vi "BundleAutoSpotData.vi"(2 "auto":bool, 3 "notes 2":refnum<vi>, 4 "already x spots":i16, 5 "Enum":enum16{"1st sort", "Display", "Get"}(ring)) -> (1 "Spots out":T1[](array[typedef]) {"F2-Value overall" format="%.2f"; "tauerror" format="%.2f"; "Lifetime[ns]" format="%.2f"; "F2-Value TAC" format="%.2f"})   [LabVIEW 2009]
uses:
  spotproperties.ctl
  <vilib>/vision/NI_Vision_Development_Module.lvlib
panel:
  in  "draw?":bool
  in  "notes":string
  out "F2-Value overall":sgl format="%.2f"
  in  "Ring":u16(ring) items=["linear y-axis", "log y-axis"]
  in  "stop":bool
  out "TAC intensity":u32[](array[numeric])
  out "overall intensity":u32[](array[numeric])
  out "tauerror [ns]":dbl[](array[numeric]) format="%.2f"
  out "Lifetime [ns]":ext[](array[numeric]) format="%.2f"
  out "F2-Value TAC":dbl format="%.2f"
  in  "SpotNo.":u16 min=1 max=74
  out "Decays":u32[][](graph)
  # "S"
  # "S"
  # "S"
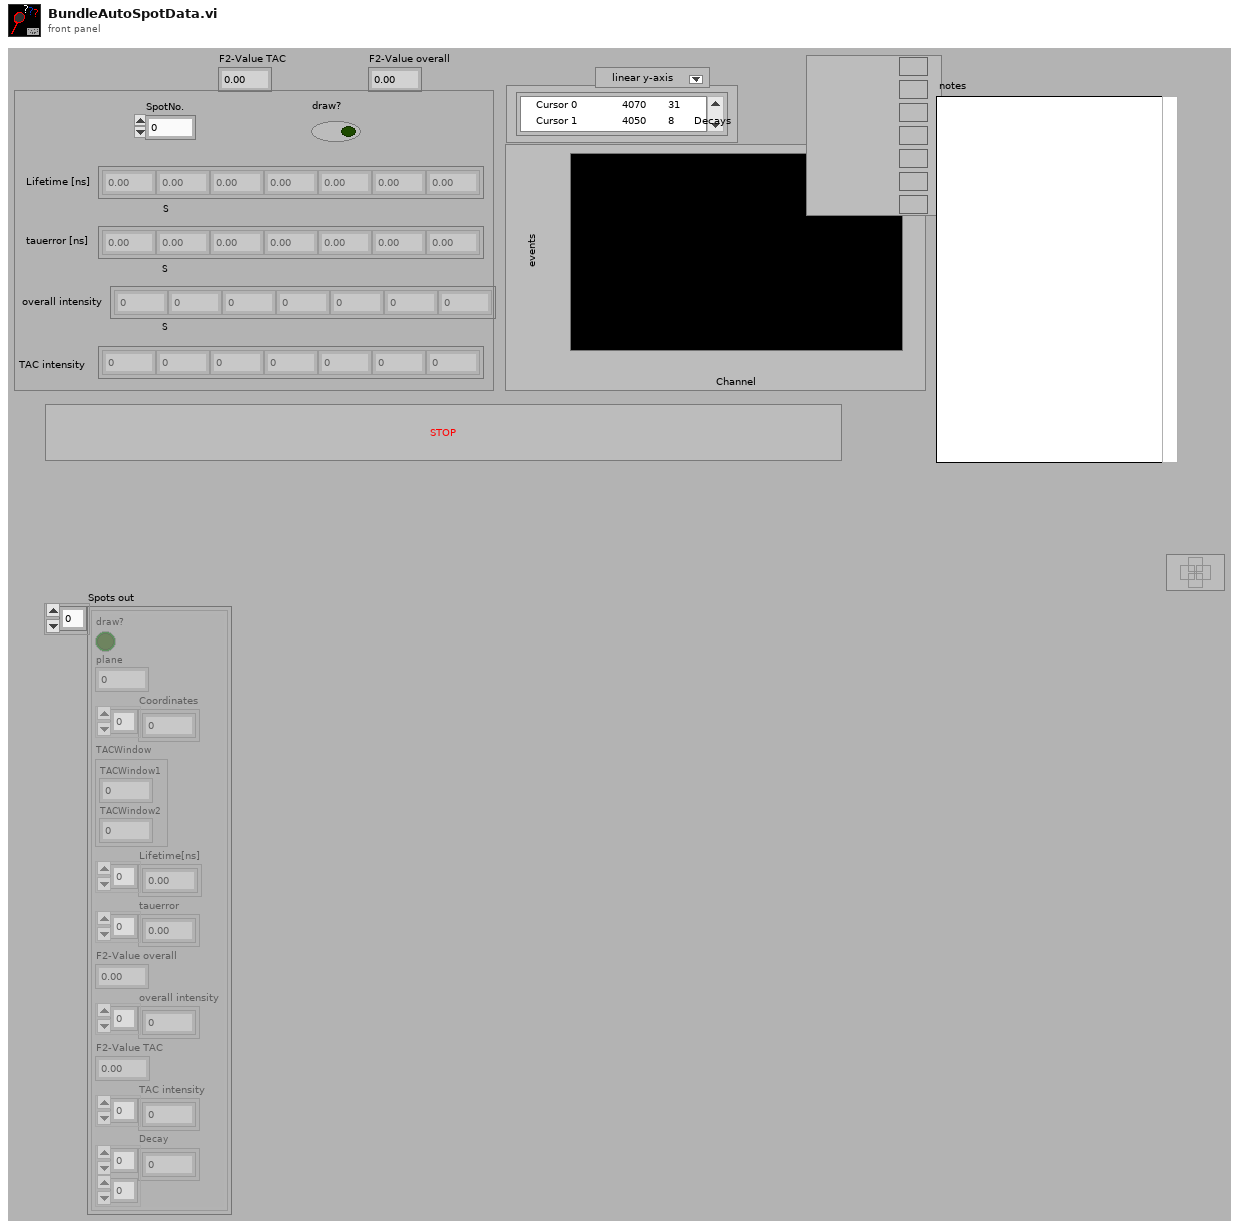
[diagram p1: front panel]
types:
  T1 = typedef "spotproperties.ctl" = cluster{"draw?":bool, "plane":u32, "Coordinates":i32[], "TACWindow":cluster{"TACWindow1":i32, "TACWindow2":i32}, "Lifetime[ns]":ext[], "tauerror":dbl[], "F2-Value overall":dbl, "overall intensity":u32[], "F2-Value TAC":dbl, "TAC intensity":u32[], "Decay":u32[][]}
  T2 = enum16{"Ini", "Get", "Set", "Refresh", "dump", "move", "name"}
  T3 = typedef "Settings.ctl" = cluster{"threshold":cluster{"max":u32, "min":u32}, "RGB or false color":bool, "16bit":bool, "log/lin axis":u16, "spotsize button":bool, "Pixelsize":u16, "autoscale x":bool, "autoscale y":bool, "correlation":bool, "ADC-Resolution":i32, "F2-lifetime":cluster{"display tau":bool, "display F2":bool, "Palette Number lifetime":enum32{"Gray", "Binary", "Gradient", "Rainbow", "Temperature"}, "Palette Number F2":enum32{"Gray", "Binary", "Gradient", "Rainbow", "Temperature"}, "max tau-Value":dbl, "min tau-Value":dbl, "max F2-Value":dbl, "min F2-Value":dbl}, "TAC-Window 1":u16, "TAC-Window 2":u16, "false color palette":cluster{"1":u32, "2":u32, "3":u32, "4":u32, "5":u32, "6":u32, "7":u32, "8":u32, "8 2":u32, "8 3":u32, "8 4":u32, "8 5":u32}, "rebinning":dbl}
  T4 = typedef "IMAQ Image.ctl" = refnum<image>
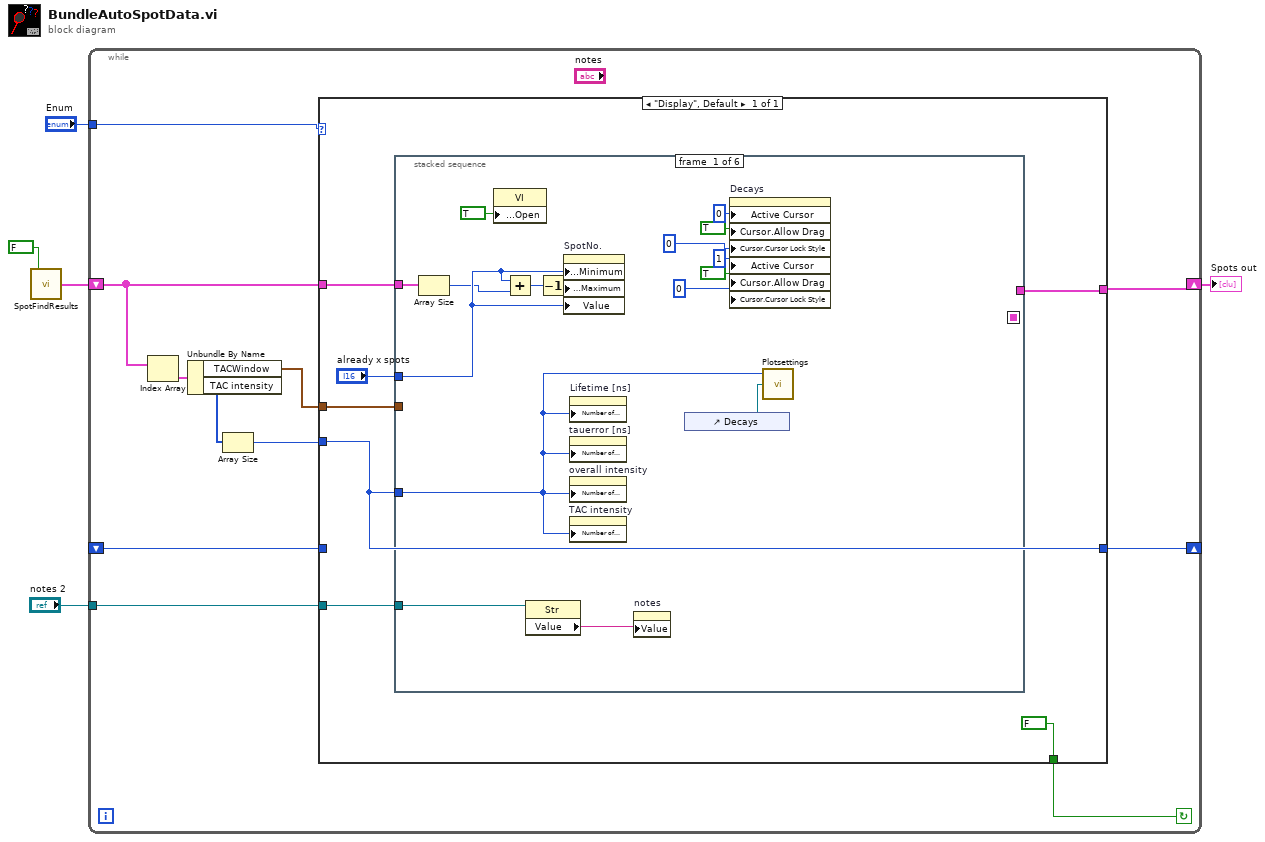
[diagram p0: block diagram]
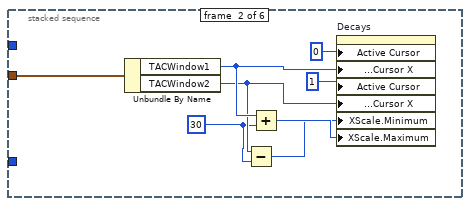
[diagram p2: hidden frame]
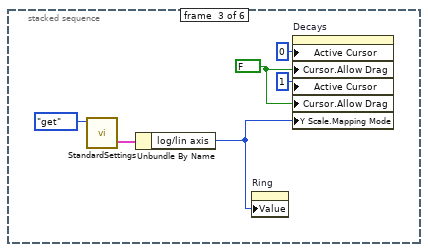
[diagram p3: hidden frame]
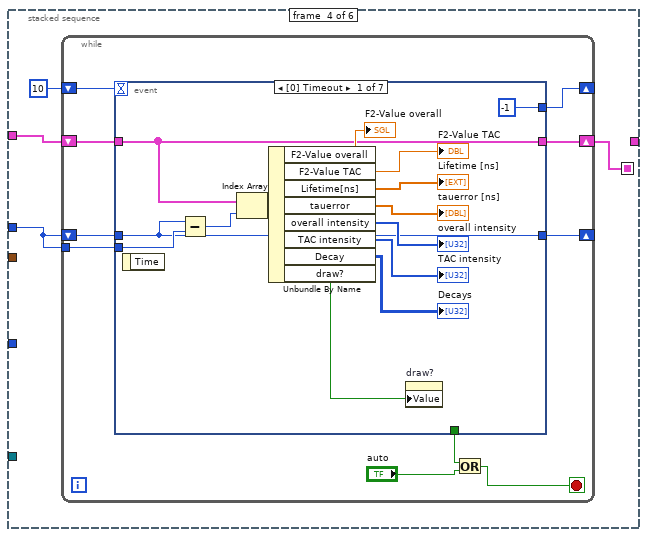
[diagram p4: hidden frame]
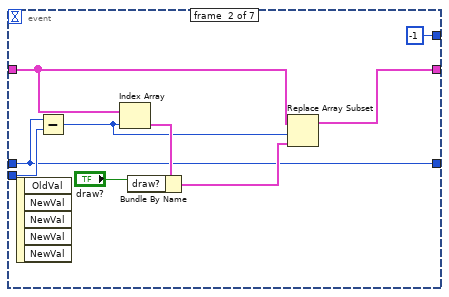
[diagram p5: hidden frame]
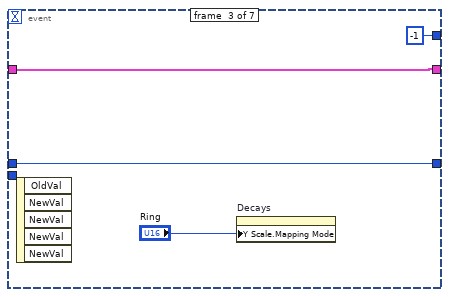
[diagram p6: hidden frame]
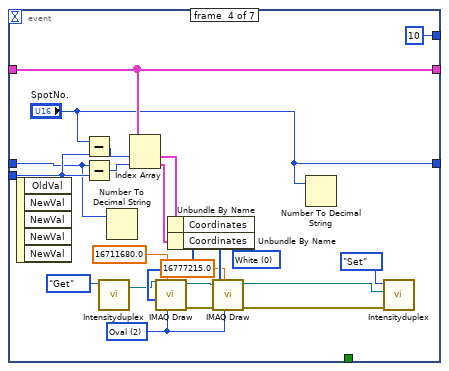
[diagram p7: hidden frame]
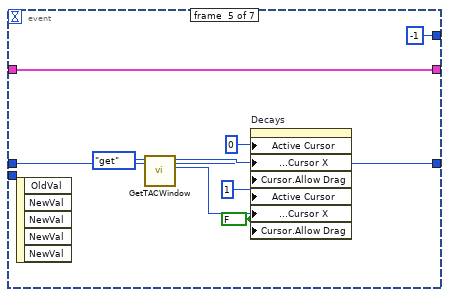
[diagram p8: hidden frame]
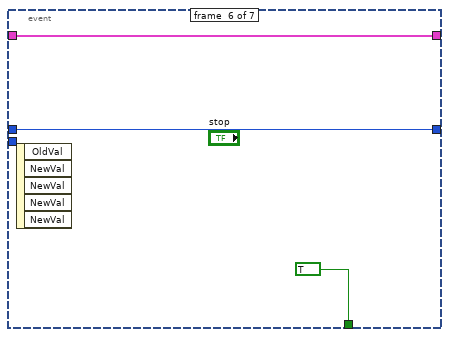
[diagram p9: hidden frame]
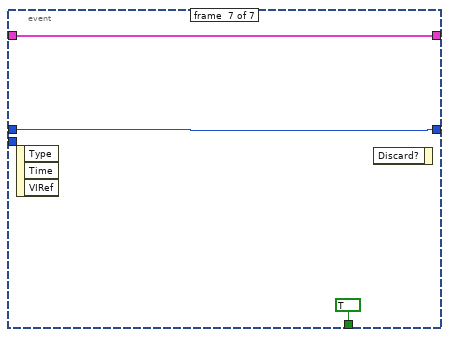
[diagram p10: hidden frame]
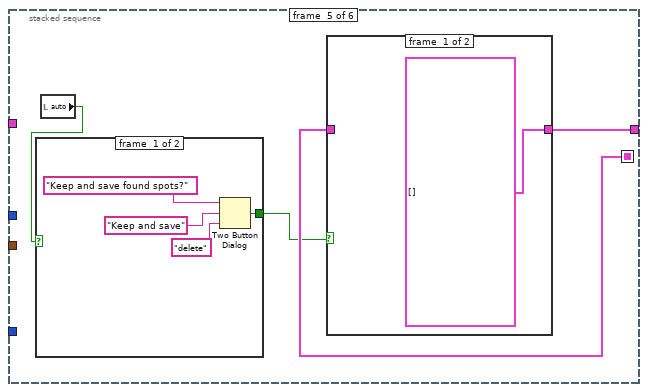
[diagram p11: hidden frame]
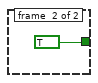
[diagram p12: hidden frame]
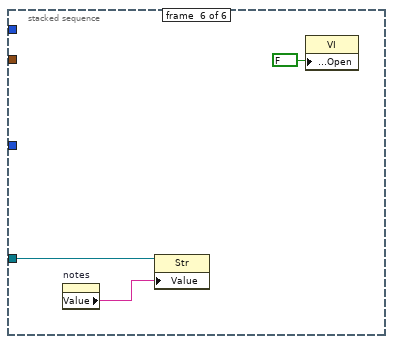
[diagram p14: hidden frame]
diagram:
  n1 = call "SpotFindResults.vi"("set?"=FALSE) -> ("Spots out"=w4:T1[])  [unwired: 4 in]
  n2 = while {
    shift-right: [w15] -> w1
    shift-left: w4 -> [w12]
    shift-right: [w14] -> _
    shift-left: _ -> [w13]
    tunnel: "Enum" -> [w7]
    tunnel: "notes 2" -> [w6]
    stop <- w16 continue-if-true
    n3 = Index Array(array=w12) -> (element=w11:T1)  [unwired: 1 in]
    n4 = Unbundle By Name(w11) -> ("TACWindow"=w10:cluster{"TACWindow1":i32, "TACWindow2":i32}, "TAC intensity"=w9:u32[])
    n5 = Array Size(array=w9) -> (size(s)=w8:i32)
    n6 = case shown="\"Display\", Default" w7 {
      tunnel: [FALSE] -> w16
      tunnel: [w22] -> w15
      tunnel: w12 -> [w23]
      tunnel: [w19] -> w14
      tunnel: w13 -> [_]
      tunnel: w10 -> [w20]
      tunnel: w8 -> [w19]
      tunnel: w6 -> [w17]
      frame "Display", Default {
        n7 = stacked-sequence {
          seq-local: [_ _ _ w55 _ _] -> [_ _ _ _ w133 _]
          tunnel: w23 -> [w38 _ _ w56 _ _]
          tunnel: [_ _ _ _ w134 _] -> w22
          tunnel: w19 -> [w28 _ _ _ _ _]
          tunnel: "already x spots" -> [w27 _ _ w54 _ _]
          tunnel: w20 -> [_ w45 _ _ _ _]
          tunnel: w17 -> [w30 _ _ _ _ w142]
          frame #0 {
            n8 = Array Size(array=w38) -> (size(s)=w26:i32)
            n9 = property class="VI"("Front Panel Window:Open"=TRUE) -> ()  [unwired: 2 in, 2 out]
            n10 = Add(x=w27, y=w26) -> (x+y=w25:i32)
            n11 = property class="Str"(reference=w30) -> ("Value"=w31:string)  [unwired: 1 in, 2 out]
            n12 = Decrement(x=w25) -> (x-1=w24:i32)
            n13 = property on="SpotNo." class="Digital (strict)"("Data Entry Limits:Minimum"=w27, "Data Entry Limits:Maximum"=w24, "Value"=w27) -> ()  [unwired: 2 in, 2 out]
            n14 = property on="Lifetime [ns]" class="Arr (strict)"("Number of Columns"=w28) -> ()  [unwired: 2 in, 2 out]
            n15 = property on="tauerror [ns]" class="Arr (strict)"("Number of Columns"=w28) -> ()  [unwired: 2 in, 2 out]
            n16 = property on="overall intensity" class="Arr (strict)"("Number of Columns"=w28) -> ()  [unwired: 2 in, 2 out]
            n17 = property on="TAC intensity" class="Arr (strict)"("Number of Columns"=w28) -> ()  [unwired: 2 in, 2 out]
            n18 = property on="notes" class="String"("Value"=w31) -> ()  [unwired: 2 in, 2 out]
            n19 = control-ref of="Decays"() -> (w29:refnum<vi>)
            n20 = property on="Decays" class="WFGraph (strict)"("Active Cursor"=u32 0, "Cursor.Allow Drag"=TRUE, "Cursor.Cursor Lock Style"=u32 0 ("Cursor.Cursor Locked"), "Active Cursor"=u32 1, "Cursor.Allow Drag"=TRUE, "Cursor.Cursor Lock Style"=u32 0 ("Cursor.Cursor Locked")) -> ()  [unwired: 2 in, 2 out]
            n21 = call "Plotsettings.vi"("Decays 2"=w29, "No of Channels"=w28) -> ()  [unwired: 4 in]
          }
          frame #1 {
            w42 = 30 ("y")
            n22 = Unbundle By Name(w45) -> ("TACWindow1"=w44:i32, "TACWindow2"=w43:i32)
            n23 = Subtract(x=w43, y=w42) -> (x-y=w40:i32)
            n24 = Add(x=w44, y=w42) -> (x+y=w41:i32)
            n25 = property on="Decays" class="WFGraph (strict)"("Active Cursor"=u32 0, "Cursor.Cursor Position:Cursor X"=w44, "Active Cursor"=u32 1, "Cursor.Cursor Position:Cursor X"=w43, "XScale.Minimum"=w40, "XScale.Maximum"=w41) -> ()  [unwired: 2 in, 2 out]
          }
          frame #2 {
            w53 = FALSE ("Cursor.Allow Drag")
            n26 = call "StandardSettings.vi"("Enum"=enum16{"Load", "get", "Save", "set"}."get") -> ("StandardSettings"=w49:T3)  [unwired: 4 in]
            n27 = Unbundle By Name(w49) -> ("log/lin axis"=w48:u16)
            n28 = property on="Ring" class="Ring (strict)"("Value"=w48) -> ()  [unwired: 2 in, 2 out]
            n29 = property on="Decays" class="WFGraph (strict)"("Active Cursor"=u32 0, "Cursor.Allow Drag"=w53, "Active Cursor"=u32 1, "Cursor.Allow Drag"=w53, "Y Scale.Mapping Mode"=w48) -> ()  [unwired: 2 in, 2 out]
          }
          frame #3 {
            n30 = while {
              shift-right: [w64] -> _
              shift-left: 10 -> [w65]
              shift-right: [w67] -> _
              shift-left: w54 -> [w66]
              shift-right: [w63] -> w55
              shift-left: w56 -> [w62]
              tunnel: w54 -> [w61]
              stop <- w58 stop-if-true
              n31 = event shown="[0] Timeout" {
                selector: _ -> [_ _ _ _ _ _ _]
                dyn-events: _ -> [_ _ _ _ _ _ _]
                timeout: w65 -> [_ _ _ _ _ _ _]
                tunnel: w62 -> [w71 w90 w92 w112 w118 w126 w129]
                tunnel: [_ _ _ _ _ TRUE TRUE] -> w60
                tunnel: [w68 w83 w91 "SpotNo." w117 w125 w128] -> w67
                tunnel: w66 -> [w68 w83 w91 w103 w117 w125 w128]
                tunnel: [-1 -1 -1 10 -1 _ _] -> w64
                tunnel: [w71 w87 w92 w112 w118 w126 w129] -> w63
                tunnel: w61 -> [w70 w84 _ w113 _ _ _]
                event #0 {
                  n32 = event-data() -> ()  [unwired: 1 in, 1 out]
                  n33 = Subtract(x=w68, y=w70) -> (x-y=w69:u16)
                  n34 = Index Array(array=w71, index=w69) -> (element=w81:T1)
                  n35 = Unbundle By Name(w81) -> ("F2-Value overall"=→"F2-Value overall":dbl, "F2-Value TAC"=→"F2-Value TAC":dbl, "Lifetime[ns]"=→"Lifetime [ns]":ext[], "tauerror"=→"tauerror [ns]":dbl[], "overall intensity"=→"overall intensity":u32[], "TAC intensity"=→"TAC intensity":u32[], "Decay"=→"Decays":u32[][], "draw?"=w72:bool)
                  n36 = property on="draw?" class="Boolean (strict)"("Value"=w72) -> ()  [unwired: 2 in, 2 out]
                }
                event #1 {
                  n37 = event-data() -> ()  [unwired: 1 in, 5 out]
                  n38 = Subtract(x=w83, y=w84) -> (x-y=w82:u16)
                  n39 = Index Array(array=w90, index=w82) -> (element=w89:T1)
                  n40 = Bundle By Name(cluster=w89, "draw?"="draw?") -> (w88:T1)
                  n41 = Replace Array Subset(array=w90, new element=w88, index=w82) -> (w87:T1[])
                }
                event #2 {
                  n42 = event-data() -> ()  [unwired: 1 in, 5 out]
                  n43 = property on="Decays" class="WFGraph (strict)"("Y Scale.Mapping Mode"="Ring") -> ()  [unwired: 2 in, 2 out]
                }
                event #3 {
                  (unwired) 0 items=["White", "Black", "Inverted", "Black on White", "White on Black"] ("Color")
                  w108 = u16 2 items=["Line", "Rectangle", "Oval"] ("Shape to draw")
                  n44 = event-data() -> ()  [unwired: 1 in, 5 out]
                  n45 = Subtract(x="SpotNo.", y=w113) -> (x-y=w111:u16)
                  n46 = Subtract(x=w103, y=w113) -> (x-y=w104:u16)
                  n47 = call "Intensityduplex.vi"("Enum"=T2."Get") -> ("Image Duplicate (out)"=w98:T4)  [unwired: 4 in, 1 out]
                  n48 = Number To Decimal String(number=w103) -> ()  [unwired: 1 in, 1 out]
                  n49 = Index Array(array=w112, index #1=w111, index #2=w104) -> (element #1=w109:T1, element #2=w110:T1)
                  n50 = Unbundle By Name(w109) -> ("Coordinates"=w105:i32[])
                  n51 = call "IMAQ Draw"("Shape to draw"=w108, "Pixel Color"=sgl 16711680.0, "Coordinates"=w105, "Image Src"=w98) -> ("error out"=w106:errorcluster, "Image Dst Out"=w97:T4)  [unwired: 6 in]
                  n52 = Unbundle By Name(w110) -> ("Coordinates"=w101:i32[])
                  n53 = call "IMAQ Draw"("Shape to draw"=w108, "Pixel Color"=sgl 16777215.0, "error in (no error)"=w106, "Coordinates"=w101, "Image Src"=w97) -> ("error out"=w95:errorcluster, "Image Dst Out"=w96:T4)  [unwired: 5 in]
                  n54 = Number To Decimal String(number="SpotNo.") -> ()  [unwired: 1 in, 1 out]
                  n55 = call "Intensityduplex.vi"("Enum"=T2."Set", "Image In"=w96, "error in"=w95) -> ()  [unwired: 2 in, 2 out]
                }
                event #4 {
                  w119 = FALSE ("Cursor.Allow Drag")
                  n56 = event-data() -> ()  [unwired: 1 in, 5 out]
                  n57 = call "GetTACWindow.vi"("Enum"=enum16{"ini", "get", "quick"}."get") -> ("Cursor.Cursor Position:Cursor X"=w123:u16, "Cursor.Cursor Position:Cursor X 2"=w122:u16)  [unwired: 1 in, 7 out]
                  n58 = property on="Decays" class="WFGraph (strict)"("Active Cursor"=u32 0, "Cursor.Cursor Position:Cursor X"=w123, "Cursor.Allow Drag"=w119, "Active Cursor"=u32 1, "Cursor.Cursor Position:Cursor X"=w122, "Cursor.Allow Drag"=w119) -> ()  [unwired: 2 in, 2 out]
                }
                event #5 {
                  n59 = event-data() -> ()  [unwired: 1 in, 5 out]
                }
                event #6 {
                  n60 = event-data() -> ()  [unwired: 1 in, 3 out]
                  n61 = event-data() -> ()  [unwired: 2 in, 1 out]
                }
              }
              n62 = Or(x=w60, y="auto") -> (x .or. y?=w58:bool)
            }
          }
          frame #4 {
            n63 = local read "auto"() -> (w131:bool)
            n64 = case shown="False" w131 {
              tunnel: [w135 TRUE] -> w132
              frame #0 {
                n65 = Two Button Dialog(message="Keep and save found spots?", 1:"delete" ("F button name (\"Cancel\")"), 2:"Keep and save" ("T button name (\"OK\")")) -> (T button?=w135:bool)
              }
              frame #1 {
              }
            }
            n66 = case shown="True" w132 {
              tunnel: w133 -> [_ w141]
              tunnel: [T1[] [] ("Spots out") w141] -> w134
              frame #0 {
              }
              frame #1 {
              }
            }
          }
          frame #5 {
            n67 = property on="notes" class="String"() -> ("Value"=w143:string)  [unwired: 2 in, 2 out]
            n68 = property class="Str"(reference=w142, "Value"=w143) -> ()  [unwired: 1 in, 2 out]
            n69 = property class="VI"("Front Panel Window:Open"=FALSE) -> ()  [unwired: 2 in, 2 out]
          }
        }
      }
    }
  }
  "Spots out" <- w1
